vi "ChannelType_2D-Array-CXT.vi"(9 "error in":errorcluster, 11 "Array in":cxt[][](array[numeric])) -> (1 "error out":errorcluster, 2 "ChannelType":ext, 3 "Array out":cxt[][](array[numeric]))   [LabVIEW 2020, in "OpenLvVision_OpenCv.lvlib"]
uses:
  OpenLvVision_OpenCv.lvlib
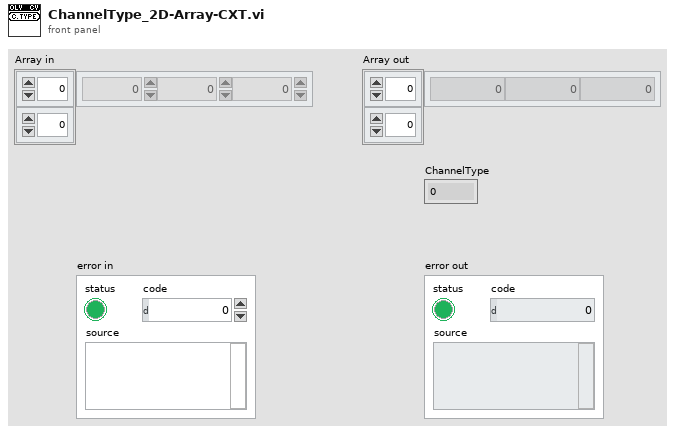
[diagram p1: front panel]
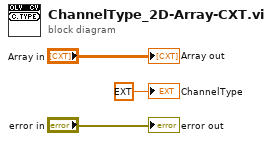
[diagram p0: block diagram]
diagram:
  "error out" <- "error in"
  "Array out" <- "Array in"
  "ChannelType" <- ext 0.0
